vi "API_GOTO.vi"(8 "error in (no error)":errorcluster, 10 "Data":dbl, 11 "Relative?":bool) -> (0 "error out":errorcluster)   [LabVIEW 2015, in "Tool Module.lvlib"]
doc: "Request the tool to move to a specified axial position or a relative distance. If the Relative? input is true, then the Data parameter specifies the distance to move from the current position. If it is false, then Data is the absolute location to move to. Units are in encoder counts."
uses:
  Tool Module.lvlib
  Support/_GoTo Cmd Typedef--enum.ctl
  Tool Config/Tool Cfg.lvlib
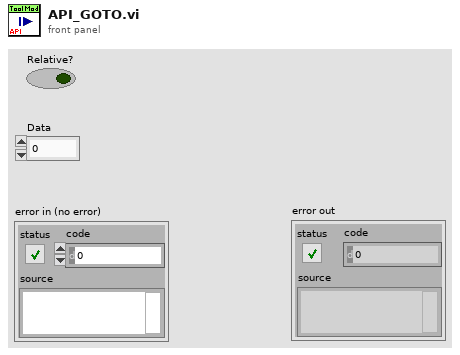
[diagram p1: front panel]
types:
  T1 = typedef "Tool Module.lvlib/_GoTo Cmd Typedef--enum.ctl" = enum16{"MoveA", "MoveR", "Home Position", "Home None", "Cleaning Position"}
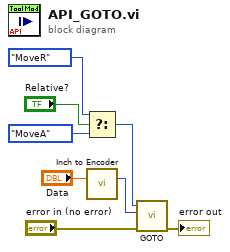
[diagram p0: block diagram]
diagram:
  n1 = Select(t=_GoTo_Cmd_Typedef--enum."MoveR" ("_GoTo Cmd typedef"), s="Relative?", f=_GoTo_Cmd_Typedef--enum."MoveA" ("_GoTo Cmd typedef")) -> (s? t:f=w6:T1)
  n2 = call "Inch to Encoder.vi"("Inches in"="Data") -> ("Encoder out"=w1:i32)  [unwired: 14 in]
  n3 = call "GOTO.vi"("error in (no error)"="error in (no error)", "Data"=w1, "GoTo Cmd"=w6) -> ("error out"=→"error out":errorcluster)  [unwired: 8 in]
